vi "Tool_Unicode Update Boolean.vi"(5 "Interpret as Unicode (T)":bool=TRUE, 6 "error in (no error)":errorcluster, 7 "Caption":string, 8 "Boolean Texts [4]":string[](array[string]), 9 "Boolean Reference":refnum<vi>) -> (0 "error out":errorcluster, 3 "Boolean Reference":refnum<vi>)   [LabVIEW 2009]
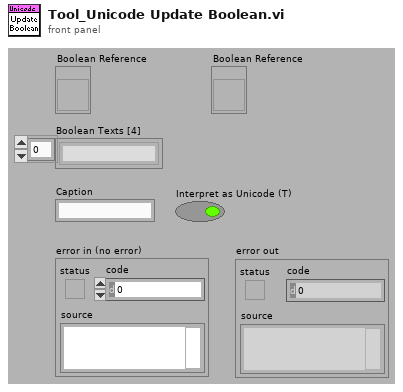
[diagram p1: front panel]
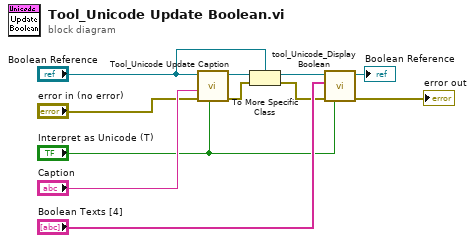
[diagram p0: block diagram]
diagram:
  n1 = call "Tool_Unicode Update Caption.vi"("Interpret as Unicode (T)"="Interpret as Unicode (T)", "error in (no error)"="error in (no error)", "Caption"="Caption", "Control Reference"="Boolean Reference") -> ("error out"=w4:errorcluster, "Control Reference"=w7:refnum<vi>)  [unwired: 4 in]
  n2 = To More Specific Class(target class="Boolean Reference", reference=w7, error in=w4) -> (specific class reference=w6:refnum<vi>, error out=w3:errorcluster)
  n3 = call "tool_Unicode_Display Boolean.vi"("Interpret as Unicode (T)"="Interpret as Unicode (T)", "error in"=w3, "Boolean Texts [4]"="Boolean Texts [4]", "Boolean Reference"=w6) -> ("error out"=→"error out":errorcluster, "Boolean Reference"=→"Boolean Reference":refnum<vi>)  [unwired: 4 in]
